vi "SettingsEditor.vi"(8 "Error In":errorcluster) -> (0 "Error Out":errorcluster)   [LabVIEW 2018]
uses:
  TraceTreeEditor/TraceTreeEditor.lvlib
  TracerLibrary/Tracer/Tracer.lvclass
panel:
  in  "Tree":string(tree) caption="Left click to select, right click to toggle activation"
  in  "Done":bool
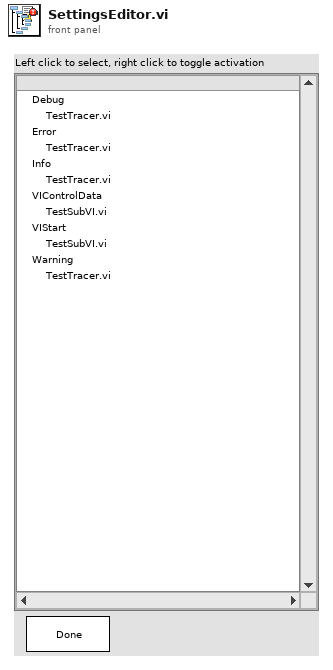
[diagram p1: front panel]
types:
  T1 = typedef "TracerLibrary.lvlib/Tracer.lvclass/TraceItemDefinition.ctl" = cluster{"Item":string, "Enable":bool}
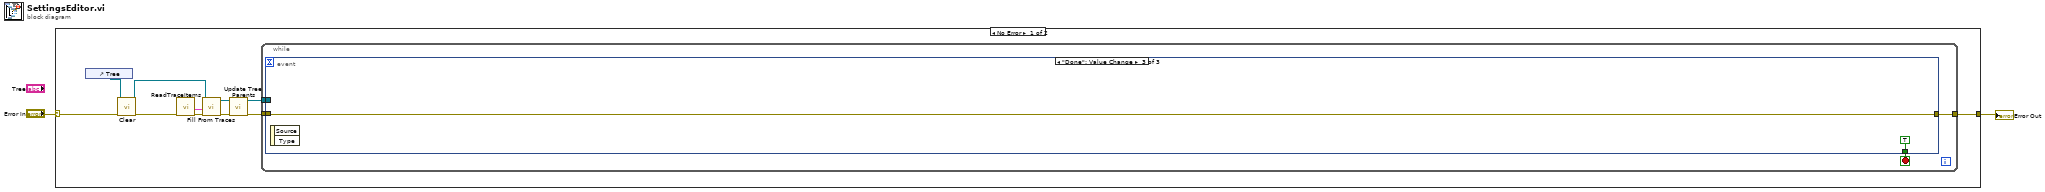
[diagram p0: block diagram]
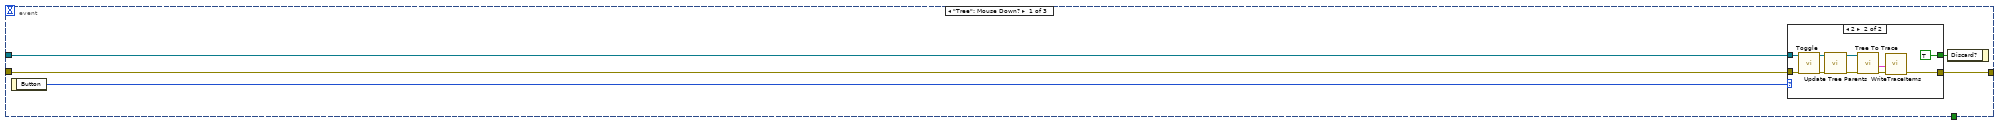
[diagram p2: hidden frame]
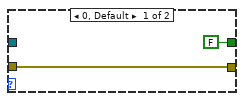
[diagram p3: hidden frame]
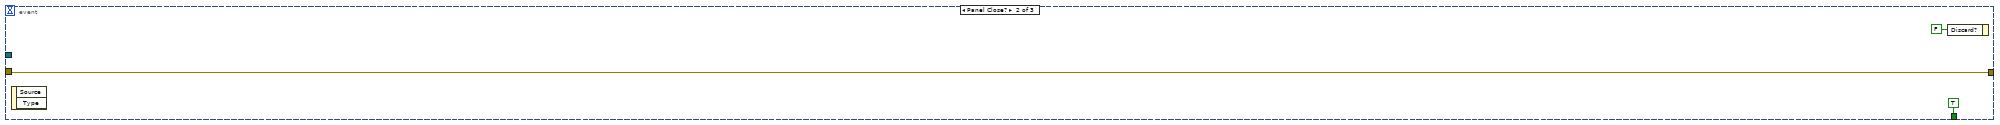
[diagram p4: hidden frame]
diagram:
  n1 = case shown="No Error" "Error In" {
    selector: "Error In" -> [w8 w40]
    tunnel: [w10 w40] -> w2
    frame No Error {
      n2 = control-ref of="Tree"() -> (w4:refnum<vi>)
      n3 = call "Clear.vi"("Error In"=w8, "Tree Control In"=w4) -> ("Error Out"=w9:errorcluster, "Tree Control Out"=w3:refnum<vi>)  [unwired: 8 in]
      n4 = call "ReadTraceItems.vi"("Error In"=w9) -> ("Error Out"=w11:errorcluster, "Trace Items"=w5:T1[])  [unwired: 9 in]
      n5 = call "Fill From Traces.vi"("Error In"=w11, "Settings"=w5, "Tree Control In"=w3) -> ("Error Out"=w13:errorcluster, "Tree Control Out"=w7:refnum<vi>)  [unwired: 7 in]
      n6 = call "Update Tree Parents.vi"("Error In"=w13, "Tree Control In"=w7) -> ("Error Out"=w12:errorcluster, "Tree Control Out"=w6:refnum<vi>)  [unwired: 8 in]
      n7 = while {
        tunnel: w6 -> [w15]
        tunnel: w12 -> [w17]
        tunnel: [w16] -> w10
        stop <- w14 stop-if-true
        n8 = event shown="[2] \"Done\": Value Change" {
          selector: _ -> [_ _ _]
          dyn-events: _ -> [_ _ _]
          timeout: _ -> [_ _ _]
          tunnel: w15 -> [w19 _ _]
          tunnel: w17 -> [w22 w37 w39]
          tunnel: [_ TRUE ("Done") TRUE ("Done")] -> w14
          tunnel: [w21 w37 w39] -> w16
          event "Tree": Mouse Down? {
            n9 = event-data() -> ("Button"=w20:u16)  [unwired: 1 in]
            n10 = case shown="2" w20 {
              tunnel: w19 -> [_ w29]
              tunnel: [FALSE ("Discard?") TRUE ("Discard?")] -> w18
              tunnel: w22 -> [w24 w31]
              tunnel: [w24 w30] -> w21
              frame 0, Default {
              }
              frame 2 {
                n11 = call "Toggle.vi"("Error In"=w31, "Tree Control In"=w29) -> ("Error Out"=w34:errorcluster, "Tree Control Out"=w27:refnum<vi>)  [unwired: 8 in]
                n12 = call "Update Tree Parents.vi"("Error In"=w34, "Tree Control In"=w27) -> ("Error Out"=w33:errorcluster, "Tree Control Out"=w26:refnum<vi>)  [unwired: 8 in]
                n13 = call "Tree To Trace.vi"("Error In"=w33, "Tree Control In"=w26) -> ("Error Out"=w32:errorcluster, "Array"=w25:cluster{string, bool}[])  [unwired: 7 in, 1 out]
                n14 = call "WriteTraceItems.vi"("Error In"=w32, "Trace Items"=w25) -> ("Error Out"=w30:errorcluster)  [unwired: 9 in]
              }
            }
            n15 = event-data("Discard?"=w18) -> ()  [unwired: 1 in, 1 out]
          }
          event Panel Close? {
            n16 = event-data() -> ()  [unwired: 1 in, 2 out]
            n17 = event-data("Discard?"=FALSE) -> ()  [unwired: 1 in, 1 out]
          }
          event "Done": Value Change {
            n18 = event-data() -> ()  [unwired: 1 in, 2 out]
          }
        }
      }
    }
    frame Error {
    }
  }
  "Error Out" <- w2
